vi "Build.vi"(8 "error in (no error)":errorcluster, 10 "Concrete Send Renamer in":refnum<class "Concrete Send Renamer.lvclass">, 11 "Scripter in":refnum<class "Message Scripter.lvclass">) -> (0 "error out":errorcluster, 2 "Concrete Send Renamer out":refnum<class "Concrete Send Renamer.lvclass">, 3 "Scripter out":refnum<class "Message Scripter.lvclass">)   [LabVIEW 2020, in "Message Maker.lvlib" / "Concrete Send Renamer.lvclass"]
uses:
  Concrete Send Renamer.lvclass
  Concrete Send Builder/Concrete Send Builder.lvclass
  Message Maker.lvlib
  Message Scripter/Message Scripter.lvclass
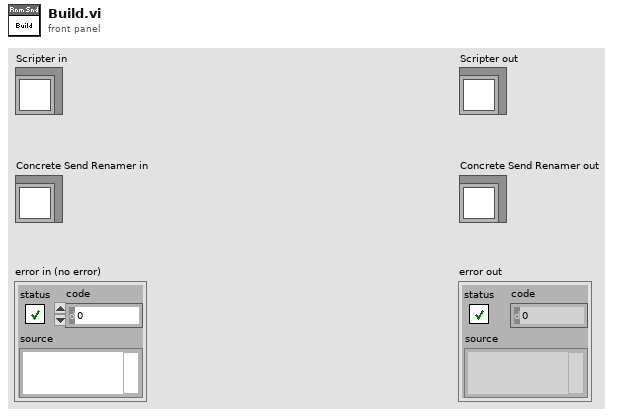
[diagram p1: front panel]
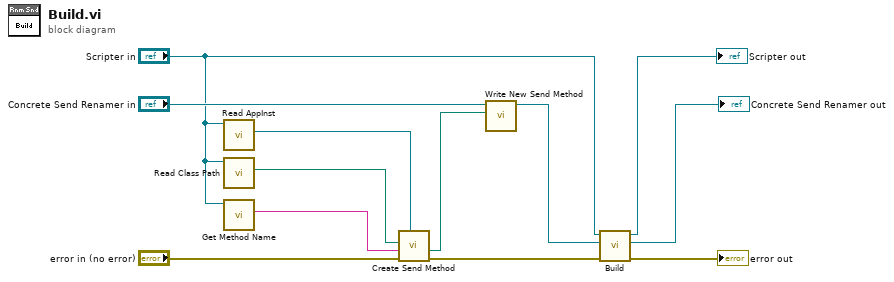
[diagram p0: block diagram]
diagram:
  n1 = call "Read AppInst.vi"("Message Maker in"="Scripter in") -> ("AppInst"=w8:refnum<vi>)  [unwired: 10 in]
  n2 = call "Read Class Path.vi"("Message Scripter in"="Scripter in") -> ("Class Path"=w9:path)  [unwired: 10 in]
  n3 = call-dynamic "Get Method Name.vi"("Message Maker in"="Scripter in") -> ("Method Name"=w1:string)  [unwired: 10 in]
  n4 = call "Create Send Method.vi"("AppInst"=w8, "error in (no error)"="error in (no error)", "Target Method"=w1, "New Class"=w9) -> ("error out"=w6:errorcluster, "New Send Method"=w3:path)  [unwired: 6 in]
  n5 = call "Write New Send Method.vi"("New Send Method"=w3, "Concrete Send Builder in"="Concrete Send Renamer in") -> ("Concrete Send Builder out"=w4:refnum<class "Concrete Send Renamer.lvclass">)  [unwired: 9 in]
  n6 = call-parent "Build.vi"("error in (no error)"=w6, "Concrete Send Builder in"=w4, "Scripter in"="Scripter in") -> ("error out"=→"error out":errorcluster, "Concrete Send Builder out"=→"Concrete Send Renamer out":refnum<class "Concrete Send Renamer.lvclass">, "Scripter out"=→"Scripter out":refnum<class "Message Scripter.lvclass">)  [unwired: 6 in]
